vi "Problem 23.vi"() -> ()   [LabVIEW 2013, in "Problem 23.lvlib"]
uses:
  Problem 23.lvlib
panel:
  out "Answer":i32
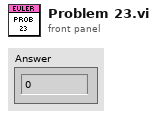
[diagram p1: front panel]
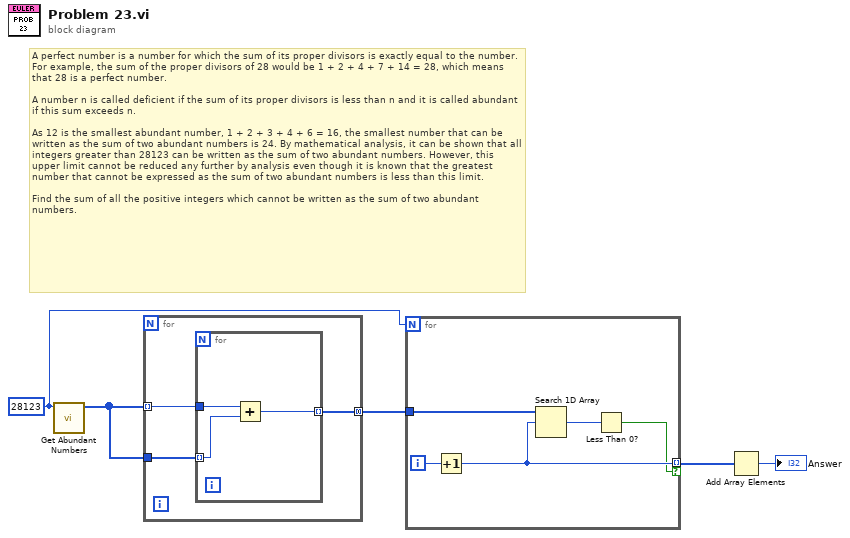
[diagram p0: block diagram]
diagram:
  w4 = 28123 ("Limit")
  # "A perfect number is a number for which the sum of its proper divisors is exactly equal to the number. For example, the sum of the proper divisors of 28 would be 1 + 2 + 4 + 7 + 14 = 28, which means that 28 is a perfect number.\n\nA number n is called deficient if the sum of its proper divisors is less than n and it is called abundant if this sum exceeds n.\n\nAs 12 is the smallest abundant number, 1 + 2 + 3 + 4 + 6 = 16, the smallest number that can be written as the sum of two abundant numbers is 24. By mathematical analysis, it can be shown that all integers greater than 28123 can be written as the sum of two abundant numbers. However, this upper limit cannot be reduced any further by analysis even though it is known that the greatest number that cannot be expressed as the sum of two abundant numbers is less than this limit.\n\nFind the sum of all the positive integers which cannot be written as the sum of two abundant numbers."
  n1 = call "Get Abundant Numbers.vi"("Limit"=w4) -> ("Abundant Numbers"=w5:i32[])  [unwired: 10 in]
  n2 = for {
    tunnel: w5 -> [w7] mode=indexing
    tunnel: w5 -> [w8]
    tunnel: [w6] -> w3 mode=concatenating
    n3 = for {
      tunnel: w8 -> [w10] mode=indexing
      tunnel: w7 -> [w11]
      tunnel: [w9] -> w6 mode=indexing
      n4 = Add(x=w11, y=w10) -> (x+y=w9:i32)
    }
  }
  n5 = for {
    N: w4 -> [_]
    tunnel: w3 -> [w15]
    tunnel: [w13] -> w2 mode=indexing if=w12
    i -> [w16]
    n6 = Increment(x=w16) -> (x+1=w13:i32)
    n7 = Search 1D Array(1D array=w15, element=w13) -> (index of element=w14:i32)  [unwired: 1 in]
    n8 = Less Than 0?(x=w14) -> (x < 0?=w12:bool)
  }
  n9 = Add Array Elements(numeric array=w2) -> (sum=→"Answer":i32)
